vi "CAM_ID_FileLoader.vi"(8 "error in":errorcluster) -> (0 "error out":errorcluster, 3 "CAM_ID":T1)   [LabVIEW 2021]
uses:
  CAM_ID.ctl
  <vilib>/Utility/xml.llb/Read From XML File(string).vi
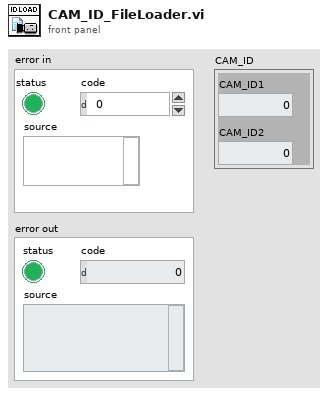
[diagram p1: front panel]
types:
  T1 = typedef "CAM_ID.ctl" = cluster{"CAM_ID1":i32, "CAM_ID2":i32}
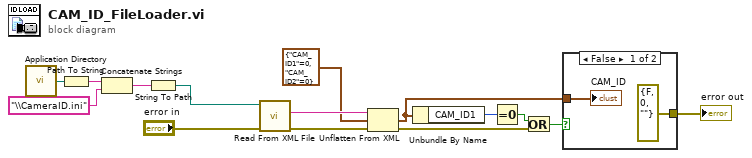
[diagram p0: block diagram]
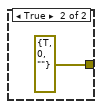
[diagram p2: hidden frame]
diagram:
  n1 = call <vilib>:"Application Directory.vi"() -> ("Application Directory"=w14:path)
  n2 = Path To String(path=w14) -> (string=w15:string)
  n3 = Concatenate Strings(w15, "\\CameraID.ini" ("string")) -> (w12:string)
  n4 = String To Path(string=w12) -> (path=w10:path)
  n5 = call-poly <vilib>:"Read From XML File.vi"("error in (no error)"="error in", "XML File Path"=w10) -> ("error out"=w8:errorcluster, "XML Elements"=w9:string)  [unwired: 7 in, 1 out]
  n6 = Unflatten From XML(xml string=w9, type=T1 {"CAM_ID1"=0, "CAM_ID2"=0} ("CAM_ID"), error in (no error)=w8) -> (value=w6:T1, error out=w3:errorcluster)
  n7 = Unbundle By Name(w6) -> ("CAM_ID1"=w7:i32)
  n8 = Equal To 0?(x=w7) -> (x = 0?=w5:bool)
  n9 = Or(x=w5, y=w3) -> (x .or. y?=w4:bool)
  n10 = case shown="False" w4 {
    tunnel: w6 -> [w17 _]
    tunnel: [errorcluster {"status"=FALSE, "code"=0, "source"=""} ("error constant") errorcluster {"status"=TRUE, "code"=0, "source"=""} ("error constant")] -> w1
    frame False {
      "CAM_ID" <- w17
    }
    frame True {
    }
  }
  "error out" <- w1
